vi "Init.vi"(9 "jettl":refnum<class "jettl.lvclass">, 10 "Self Alias":string) -> (3 "Create Msg Strategy out":refnum<class "Create Msg Strategy.lvclass">)   [LabVIEW 2021, in "Create Msg Strategy.lvlib" / "Create Msg Strategy.lvclass"]
uses:
  Create Msg Strategy.lvclass
  Create Msg Strategy.lvclass/Create Msg Strategy.ctl
  jettl/jettl/jettl.lvclass
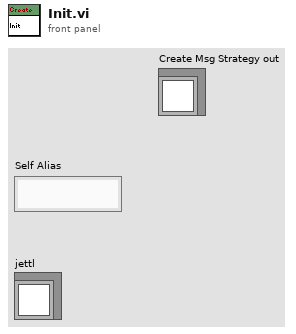
[diagram p1: front panel]
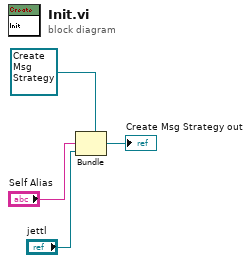
[diagram p0: block diagram]
diagram:
  n1 = Bundle "Bundle"(cluster=refnum<class "Create Msg Strategy.lvclass"> refnum ("Create Msg in"), "Self Alias", "jettl") -> (→"Create Msg Strategy out":refnum<class "Create Msg Strategy.lvclass">)  [unwired: 1 in]
